vi "PH_PP_CurrentMeas.PC _Sequencer SM State.vi"(0 "i ref in":refnum<vi>, 2 "Sequencer SM State":string, 5 "error in (no error)":errorcluster) -> (14 "i ref out":refnum<vi>, 19 "error out":errorcluster)   [LabVIEW 2014, in "PH_PP_CurrentMeas.lvlib"]
uses:
  PH_PP_CurrentMeas.lvlib
  PH_Common/PH_Common.lvlib
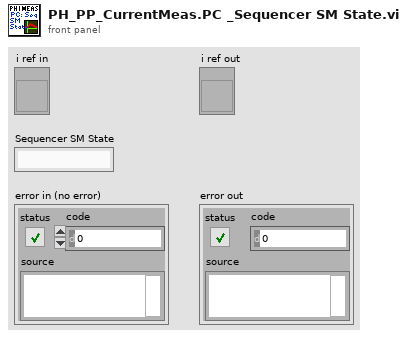
[diagram p1: front panel]
types:
  T1 = typedef "PH_PP_CurrentMeas.lvlib/PH_PP_CurrentMeas.i attribute.ctl" = cluster{"Status":cluster{"GUI Ref Hardware Feedback":refnum<vi>, "Tab Control":refnum<vi>}, "PU 1":cluster{"Instance":string, "Status":T2, "Ref Status ":refnum<vi>, "Data":waveform(dbl)[], "Ref Data":refnum<vi>}, "PU 2":cluster{"Instance":string, "Status":T2, "Ref Status ":refnum<vi>, "Data":waveform(dbl)[], "Ref Data":refnum<vi>}, "PU 3":cluster{"Instance":string, "Status":T2, "Ref Status ":refnum<vi>, "Data":waveform(dbl)[], "Ref Data":refnum<vi>}, "PU 4":cluster{"Instance":string, "Status":T2, "Ref Status ":refnum<vi>, "Data":waveform(dbl)[], "Ref Data":refnum<vi>}, "PU 5":cluster{"Instance":string, "Status":T2, "Ref Status ":refnum<vi>, "Data":waveform(dbl)[], "Ref Data":refnum<vi>}, "FR":cluster{"Instance":string, "Status":T2, "Ref Status ":refnum<vi>, "Data":waveform(dbl)[], "Ref Data":refnum<vi>}, "PA - 19mm 1":cluster{"Instance":string, "Status":T2, "Ref Status ":refnum<vi>}, "PA - 19mm 2":cluster{"Instance":string, "Status":T2, "Ref Status ":refnum<vi>, "no link":bool}, "PA - 45mm":cluster{"Instance":string, "Status":T2, "Ref Status ":refnum<vi>, "no link":bool}, "PA Data":cluster{"Data":waveform(dbl)[], "Ref":refnum<vi>}, "Sequencer":cluster{"Instance":string, "SM State Ref":refnum<vi>}, "Tasks":cluster{"Port":u16, "connection ID":refnum<k5>, "Status":T2, "Ref":refnum<vi>, "Ref Bar":refnum<vi>, "Feedback":cluster{"Received Data Sets":T3[], "Driver Error":errorcluster, "Connection not established":bool, "Error unpacking the data":bool, "No Task defined":bool, "Not triggered yet":bool}, "Data":waveform(dbl)[], "Ref Teststart Task":refnum<vi>}[], "in use":cluster{"MA DP":bool, "FR and PA":bool}, "DAQ Server":string}
  T2 = typedef "PH_StatusHandler.lvlib/PH_StatusHandler.Status.ctl" = i16
  T3 = typedef "PH_PP_CurrentMeas.lvlib/PH_PP_CurrentMeas.CommandCluster.ctl" = cluster{"Command":string, "Data":string, "error out":errorcluster}
  T4 = cluster{"Port":u16, "connection ID":refnum<k5>, "Status":T2, "Ref":refnum<vi>, "Ref Bar":refnum<vi>, "Feedback":cluster{"Received Data Sets":T3[], "Driver Error":errorcluster, "Connection not established":bool, "Error unpacking the data":bool, "No Task defined":bool, "Not triggered yet":bool}, "Data":waveform(dbl)[], "Ref Teststart Task":refnum<vi>}[]
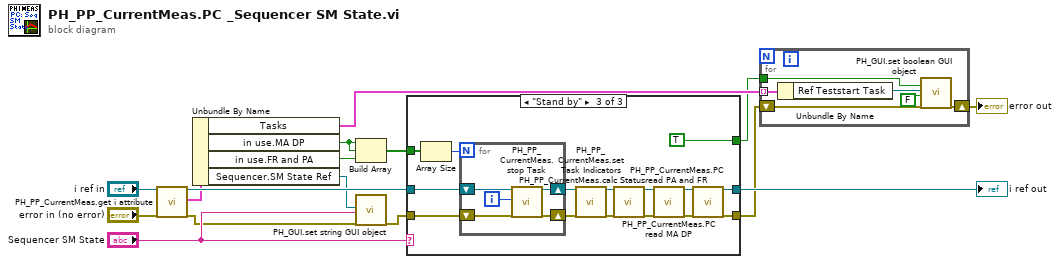
[diagram p0: block diagram]
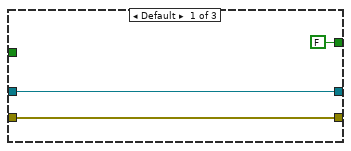
[diagram p2: hidden frame]
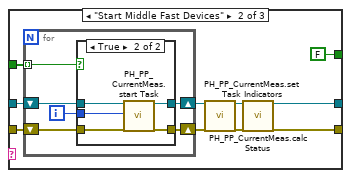
[diagram p3: hidden frame]
diagram:
  n1 = call "PH_PP_CurrentMeas.get i attribute.vi"("i ref in"="i ref in", "error in (no error)"="error in (no error)") -> ("i ref out"=w14:refnum<vi>, "i attribute"=w8:T1, "error out"=w11:errorcluster)  [unwired: 15 in]
  n2 = Unbundle By Name(w8) -> ("Tasks"=w2:T4, "in use.MA DP"=w6:bool, "in use.FR and PA"=w5:bool, "Sequencer.SM State Ref"=w4:refnum<vi>)
  n3 = Build Array(w6, w6, w5) -> (w7:bool[])
  n4 = call "PH_GUI.set string GUI object.vi"("GUI object Ref"=w4, "Text"="Sequencer SM State", "error in"=w11) -> ("error out"=w13:errorcluster)  [unwired: 16 in]
  n5 = case shown="\"Stand by\"" "Sequencer SM State" {
    tunnel: [w18 w23 w47] -> w12
    tunnel: w13 -> [w18 w21 w52]
    tunnel: w14 -> [w19 w22 w53]
    tunnel: [w19 w25 w46] -> w15
    tunnel: w7 -> [_ w29 w44]
    tunnel: [FALSE ("Visible (true)") FALSE ("Visible (true)") TRUE ("Visible (true)")] -> w1
    frame Default {
    }
    frame "Start Middle Fast Devices" {
      n6 = for {
        shift-right: [w32] -> w28
        shift-left: w21 -> [w33]
        shift-right: [w34] -> w27
        shift-left: w22 -> [w35]
        tunnel: w29 -> [w30] mode=indexing
        i -> [w31]
        n7 = case shown="True" w30 {
          tunnel: w35 -> [w37 w39]
          tunnel: [w37 w42] -> w34
          tunnel: w33 -> [w36 w38]
          tunnel: [w36 w41] -> w32
          tunnel: w31 -> [_ w40]
          frame False {
          }
          frame True {
            n8 = call "PH_PP_CurrentMeas.start Task.vi"("i ref in"=w39, "Task #"=w40, "error in (no error)"=w38) -> ("i ref out"=w42:refnum<vi>, "error out"=w41:errorcluster)  [unwired: 15 in]
          }
        }
      }
      n9 = call "PH_PP_CurrentMeas.set Task Indicators.vi"("i ref in"=w27, "error in (no error)"=w28) -> ("i ref out"=w26:refnum<vi>, "error out"=w24:errorcluster)  [unwired: 16 in]
      n10 = call "PH_PP_CurrentMeas.calc Status.vi"("i ref in"=w26, "error in (no error)"=w24) -> ("i ref out"=w25:refnum<vi>, "error out"=w23:errorcluster)  [unwired: 16 in]
    }
    frame "Stand by" {
      n11 = Array Size(array=w44) -> (size(s)=w51:i32)
      n12 = for {
        N: w51 -> [_]
        shift-right: [w61] -> w57
        shift-left: w52 -> [w58]
        shift-right: [w62] -> w56
        shift-left: w53 -> [w59]
        i -> [w60]
        n13 = call "PH_PP_CurrentMeas.stop Task.vi"("i ref in"=w59, "Task #"=w60, "error in (no error)"=w58) -> ("i ref out"=w62:refnum<vi>, "error out"=w61:errorcluster)  [unwired: 15 in]
      }
      n14 = call "PH_PP_CurrentMeas.set Task Indicators.vi"("i ref in"=w56, "error in (no error)"=w57) -> ("i ref out"=w55:refnum<vi>, "error out"=w54:errorcluster)  [unwired: 16 in]
      n15 = call "PH_PP_CurrentMeas.calc Status.vi"("i ref in"=w55, "error in (no error)"=w54) -> ("i ref out"=w50:refnum<vi>, "error out"=w48:errorcluster)  [unwired: 16 in]
      n16 = call "PH_PP_CurrentMeas.PC read MA DP.vi"("i ref in"=w50, "error in (no error)"=w48) -> ("i ref out"=w45:refnum<vi>, "error out"=w49:errorcluster)  [unwired: 16 in]
      n17 = call "PH_PP_CurrentMeas.PC read PA and FR.vi"("i ref in"=w45, "error in (no error)"=w49) -> ("i ref out"=w46:refnum<vi>, "error out"=w47:errorcluster)  [unwired: 16 in]
    }
  }
  "i ref out" <- w15
  n18 = for {
    shift-right: [w68] -> w3
    shift-left: w12 -> [w66]
    tunnel: w2 -> [w67] mode=indexing
    tunnel: w1 -> [w63]
    n19 = Unbundle By Name(w67) -> ("Ref Teststart Task"=w65:refnum<vi>)
    n20 = call "PH_GUI.set boolean GUI object.vi"("Visible (true)"=w63, "Boolean Knob GUI Ref"=w65, "Value"=FALSE, "error in (no error)"=w66) -> ("error out"=w68:errorcluster)  [unwired: 15 in]
  }
  "error out" <- w3
